vi "Find Endpoint Aliases and Routing Channels Sections.vi"(8 "error in":errorcluster, 11 "routing and faulting custom device in":T1 format="%.0x") -> (0 "error out":errorcluster, 1 "routing channels":T1 format="%.0x", 2 "endpoint aliases":T1 format="%.0x", 3 "routing and faulting custom device out":T1 format="%.0x")   [LabVIEW 2020, in "Routing and Faulting Scripting.lvlib"]
doc: "Returns the Endpoint Aliases and Routing Channels sections for the custom device."
uses:
  Routing and Faulting Scripting.lvlib
  <vilib>/NI VeriStand/Custom Device API/Custom Device Item Ref.ctl
  NationalInstruments.VeriStand.SystemDefinitionAPI
  Shared/Constants.vi
  Shared/Routing and Faulting Shared.lvlib
  <vilib>/NI VeriStand/Custom Device API/Custom Device API.lvlib
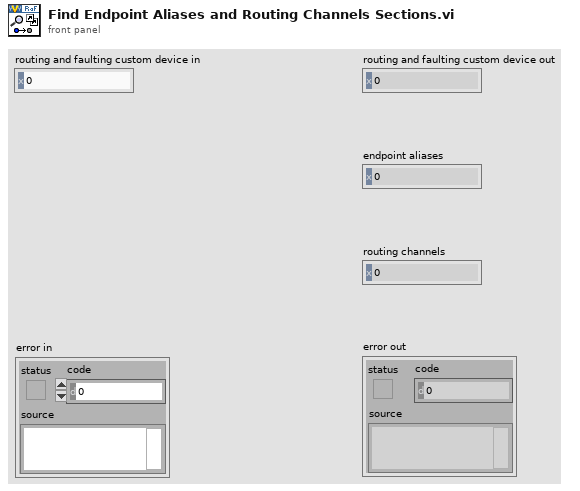
[diagram p1: front panel]
types:
  T1 = typedef "Custom Device API.lvlib/Custom Device Item Ref.ctl" = u64
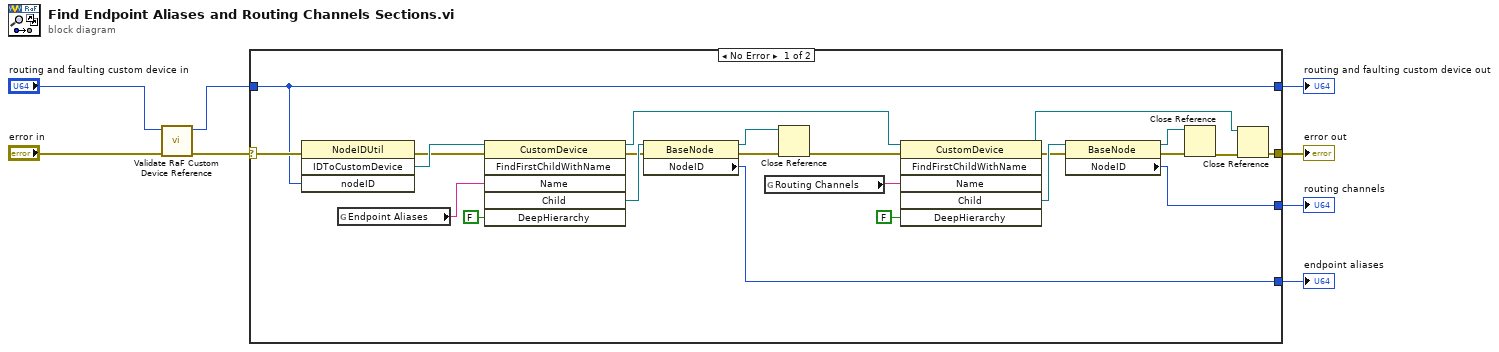
[diagram p0: block diagram]
diagram:
  n1 = call "Validate RaF Custom Device Reference.vi"("error in"="error in", "routing and faulting in"="routing and faulting custom device in") -> ("error out"=w1:errorcluster, "routing and faulting out"=w3:T1)  [unwired: 8 in]
  n2 = case shown="No Error" w1 {
    selector: w1 -> [w21 w33]
    tunnel: w3 -> [w13 w32]
    tunnel: [w13 w32] -> w8
    tunnel: [w27 _] -> w7
    tunnel: [w14 w33] -> w6
    tunnel: [w11 _] -> w5
    frame No Error {
      n3 = invoke class="NodeIDUtil" method="IDToCustomDevice"(error in=w21, "nodeID"=w13) -> (error out=w20:errorcluster, "IDToCustomDevice"=w22:refnum<k24>)  [unwired: 2 in, 2 out]
      n4 = global read "Constants.vi" "Endpoint Aliases"() -> (w12:string)
      n5 = invoke class="CustomDevice" method="FindFirstChildWithName"(reference=w22, error in=w20, "Name"=w12, "DeepHierarchy"=FALSE) -> (reference out=w16:refnum<k24>, error out=w29:errorcluster, "Child"=w31:refnum<k24>)  [unwired: 2 in, 3 out]
      n6 = property class="BaseNode"(reference=w31, error in=w29) -> (reference out=w18:refnum<k24>, error out=w19:errorcluster, "NodeID"=w11:u64)
      n7 = global read "Constants.vi" "Routing Channels"() -> (w10:string)
      n8 = Close Reference(reference=w18, error in (no error)=w19) -> (error out=w17:errorcluster)
      n9 = invoke class="CustomDevice" method="FindFirstChildWithName"(reference=w16, error in=w17, "Name"=w10, "DeepHierarchy"=FALSE) -> (reference out=w9:refnum<k24>, error out=w28:errorcluster, "Child"=w30:refnum<k24>)  [unwired: 2 in, 3 out]
      n10 = property class="BaseNode"(reference=w30, error in=w28) -> (reference out=w23:refnum<k24>, error out=w24:errorcluster, "NodeID"=w27:u64)
      n11 = Close Reference(reference=w23, error in (no error)=w24) -> (error out=w15:errorcluster)
      n12 = Close Reference(reference=w9, error in (no error)=w15) -> (error out=w14:errorcluster)
    }
    frame Error {
    }
  }
  "routing and faulting custom device out" <- w8
  "endpoint aliases" <- w5
  "routing channels" <- w7
  "error out" <- w6
